vi "Message to Byte Array.vi"(0 "Input Data":T1 {"Command" format="%02x"; "Destination" format="%02x"; "Source" format="%02x"}, 11 "Error In":errorcluster) -> (4 "Byte Array":u8[](array[numeric]), 15 "Error Out":errorcluster)   [LabVIEW 2019, in "GEA2_Toolkit.lvlib"]
uses:
  library/GEA2_Toolkit.lvlib
  type defs/Data In.ctl
  C:/TechnologyLab/NI-2010/Drivers/GEA3 Toolkit/GEA3 DLL Source/Utilities.dll
  GEA3 DLL Source/Utilities.dll
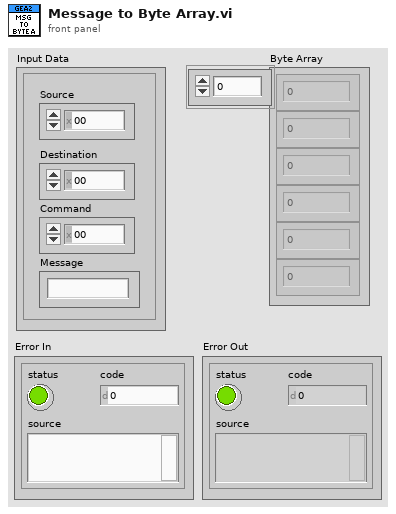
[diagram p1: front panel]
types:
  T1 = typedef "GEA2_Toolkit.lvlib/Data In.ctl" = cluster{"Source":u8, "Destination":u8, "Command":u8, "Message":string}
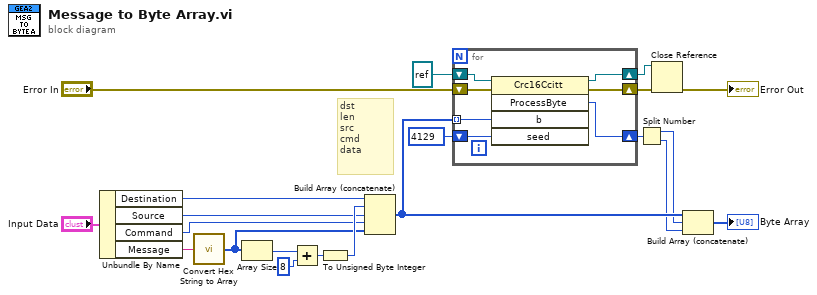
[diagram p0: block diagram]
diagram:
  # "dst\nlen\nsrc\ncmd\ndata"
  n1 = Unbundle By Name("Input Data") -> ("Destination"=w16:u8, "Source"=w17:u8, "Command"=w18:u8, "Message"=w15:string)
  n2 = call "Convert Hex String to Array.vi"("Hex String In"=w15) -> ("Hex Array Out"=w12:u8[])  [unwired: 14 in]
  n3 = Array Size(array=w12) -> (size(s)=w13:i32)
  n4 = Add(x=w13, y=8) -> (x+y=w20:i32)
  n5 = To Unsigned Byte Integer(number=w20) -> (unsigned 8bit integer=w19:u8)
  n6 = Build Array (concatenate)(w16, w19, w17, w18, w12) -> (w4:u8[])
  n7 = for {
    tunnel: w4 -> [w28] mode=indexing
    shift-right: [w26] -> w10
    shift-left: u16 4129 ("seed") -> [w27]
    shift-right: [w24] -> w8
    shift-left: "Error In" -> [w25]
    shift-right: [w22] -> w7
    shift-left: refnum<k24> refnum ("reference") -> [w23]
    n8 = invoke class="Crc16Ccitt" method="ProcessByte"(reference=w23, error in=w25, "b"=w28, "seed"=w27) -> (reference out=w22:refnum<k24>, error out=w24:errorcluster, "ProcessByte"=w26:u16)  [unwired: 1 in, 2 out]
  }
  n9 = Split Number(x=w10) -> (hi(x)=w2:u8, lo(x)=w3:u8)
  n10 = Close Reference(reference=w7, error in (no error)=w8) -> (error out=→"Error Out":errorcluster)
  n11 = Build Array (concatenate)(w4, w2, w3) -> (→"Byte Array":u8[])
